vi "add tag to table.vi"(8 "error in":errorcluster, 10 "system tag":refnum<class "tag descriptor.lvclass">, 11 "data table in":T1) -> (0 "error out":errorcluster, 3 "data table out":T1)   [LabVIEW 2013, in "tag bus.lvlib" / "data table.lvlib"]
doc: "Adds a tag to a data table."
uses:
  data table.lvlib
  data table.ctl
  tag/tag descriptor.lvclass
  tag/tag descriptor.lvclass/tag descriptor.ctl
  tag/default value polymorphs/read default value Double.vi
  tag/default value polymorphs/read default value Single.vi
  tag/default value polymorphs/read default value I64.vi
  tag/default value polymorphs/read default value I32.vi
  tag/default value polymorphs/read default value I16.vi
  tag/default value polymorphs/read default value I8.vi
  tag/default value polymorphs/read default value U64.vi
  tag/default value polymorphs/read default value U32.vi
  tag/default value polymorphs/read default value U16.vi
  tag/default value polymorphs/read default value U8.vi
  tag/default value polymorphs/read default value String.vi
  tag/default value polymorphs/read default value Boolean.vi
  tag/default value polymorphs/read default value Array of U8.vi
  tag/default value polymorphs/read default value Array of U16.vi
  tag/default value polymorphs/read default value Array of U32.vi
  tag/default value polymorphs/read default value Array of U64.vi
  tag/default value polymorphs/read default value Array of I64.vi
  tag/default value polymorphs/read default value Array of I32.vi
  tag/default value polymorphs/read default value Array of I16.vi
  tag/default value polymorphs/read default value Array of I8.vi
  tag/default value polymorphs/read default value Array of Double.vi
  tag/default value polymorphs/read default value Array of Single.vi
  tag/default value polymorphs/read default value Array of Boolean.vi
  tag/default value polymorphs/read default value Array of String.vi
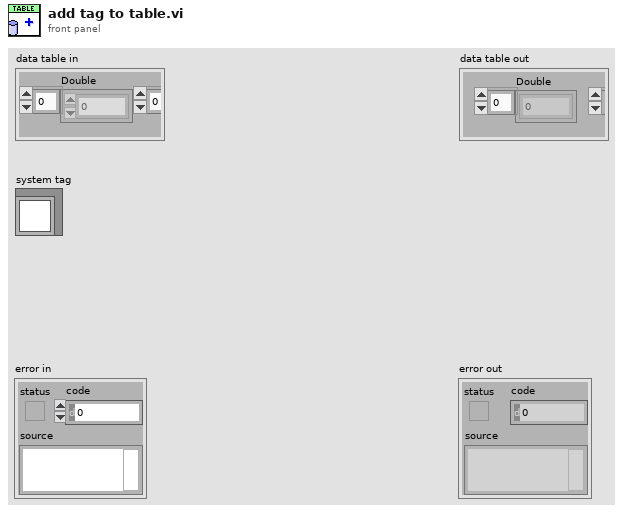
[diagram p1: front panel]
types:
  T1 = typedef "tag bus.lvlib/data table.lvlib/data table.ctl" = cluster{"Double":dbl[], "Single":sgl[], "I64":i64[], "I32":i32[], "I16":i16[], "I8":i8[], "U64":u64[], "U32":u32[], "U16":u16[], "U8":u8[], "Boolean":bool[], "String":string[], "Array of Double":cluster{"DBL Array":dbl[]}[], "Array of Single":cluster{"SGL Array":sgl[]}[], "Array of I64":cluster{"I64 Array":i64[]}[], "Array of I32":cluster{"I32 Array":i32[]}[], "Array of I16":cluster{"I16 Array":i16[]}[], "Array of I8":cluster{"I8 Array":i8[]}[], "Array of U64":cluster{"U64 Array":u64[]}[], "Array of U32":cluster{"U32 Array":u32[]}[], "Array of U16":cluster{"U16 Array":u16[]}[], "Array of U8":cluster{"U8 Array":u8[]}[], "Array of Boolean":cluster{"Boolean Array":bool[]}[], "Array of String":cluster{"String Array":string[]}[]}
  T2 = typedef "tag bus.lvlib/tag descriptor.lvclass/Data Type.ctl" = enum16{"Double", "Single", "I64", "I32", "I16", "I8", "U64", "U32", "U16", "U8", "Boolean", "String", "Array of Double", "Array of Single", "Array of I64", "Array of I32", "Array of I16", "Array of I8", "Array of U64", "Array of U32", "Array of U16", "Array of U8", "Array of Boolean", "Array of String"}
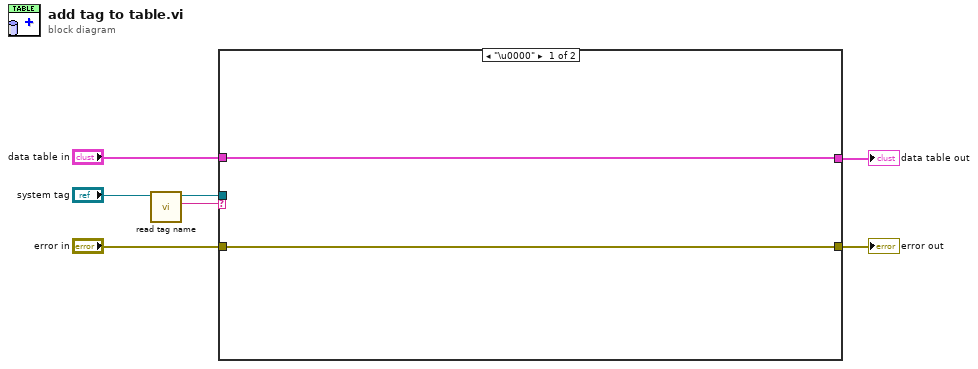
[diagram p0: block diagram]
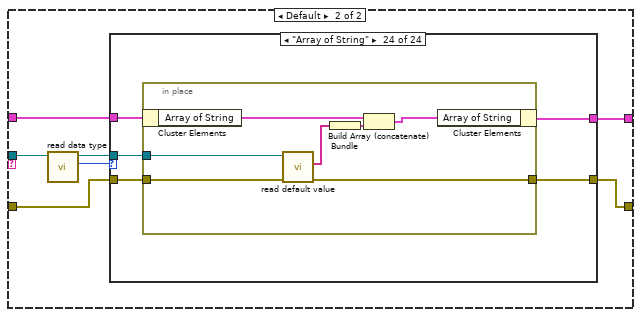
[diagram p2: hidden frame]
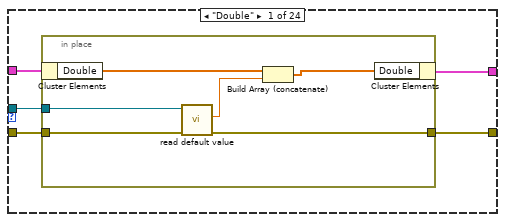
[diagram p3: hidden frame]
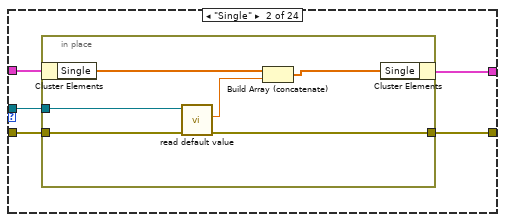
[diagram p4: hidden frame]
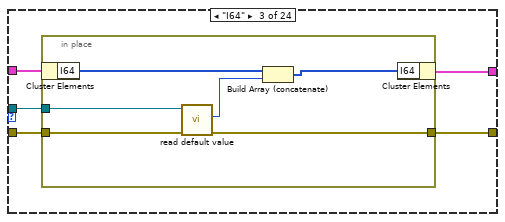
[diagram p5: hidden frame]
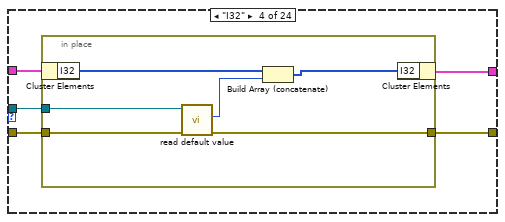
[diagram p6: hidden frame]
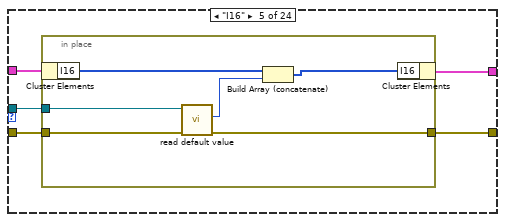
[diagram p7: hidden frame]
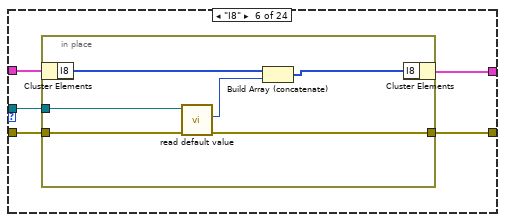
[diagram p8: hidden frame]
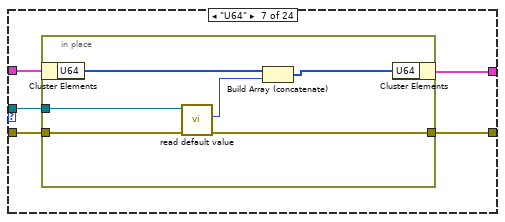
[diagram p9: hidden frame]
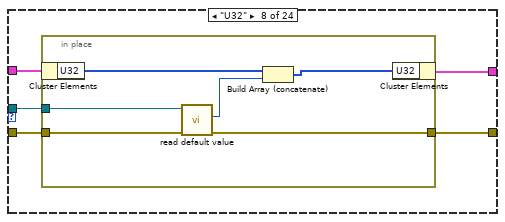
[diagram p10: hidden frame]
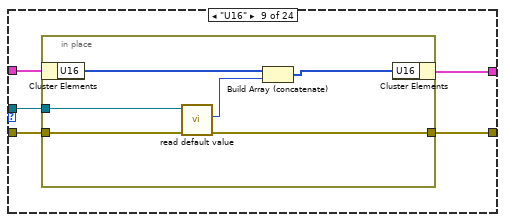
[diagram p11: hidden frame]
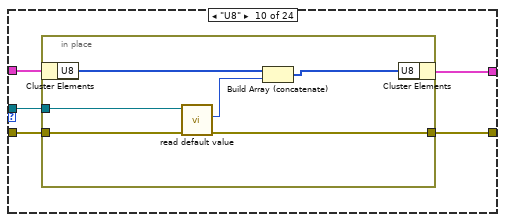
[diagram p12: hidden frame]
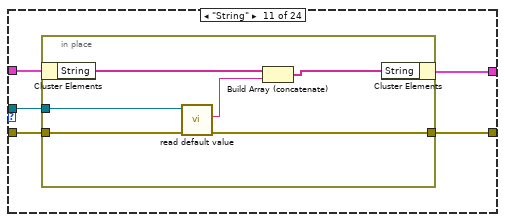
[diagram p13: hidden frame]
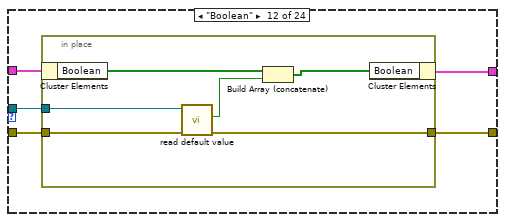
[diagram p14: hidden frame]
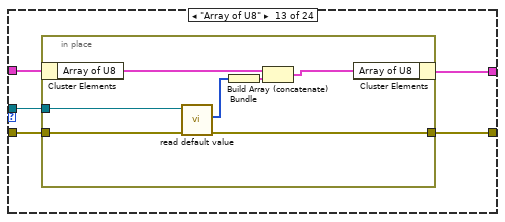
[diagram p15: hidden frame]
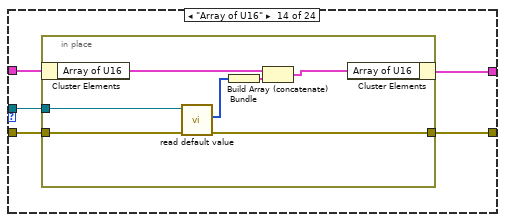
[diagram p16: hidden frame]
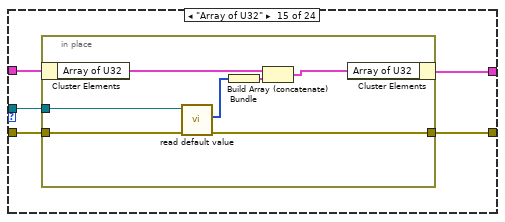
[diagram p17: hidden frame]
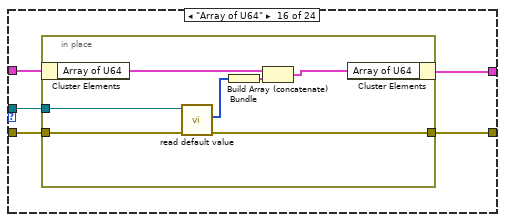
[diagram p18: hidden frame]
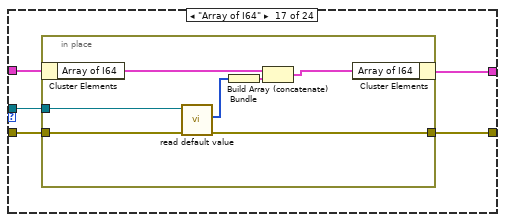
[diagram p19: hidden frame]
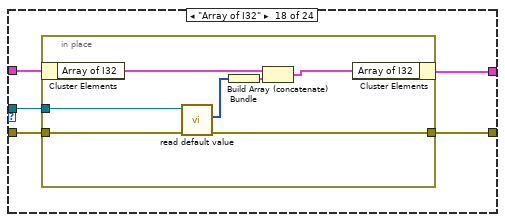
[diagram p20: hidden frame]
diagram:
  n1 = call "read tag name.vi"("system tag in"="system tag") -> ("name"=w1:string, "system tag out"=w2:refnum<class "tag descriptor.lvclass">)  [unwired: 8 in, 1 out]
  n2 = case shown="\"\"" w1 {
    tunnel: "data table in" -> [w9 w15]
    tunnel: [w9 w14] -> w6
    tunnel: "error in" -> [w8 w12]
    tunnel: [w8 w11] -> w4
    tunnel: w2 -> [_ w10]
    frame "\u0000" {
    }
    frame Default {
      n3 = call "read data type.vi"("system tag in"=w10) -> ("data type"=w16:T2, "system tag out"=w13:refnum<class "tag descriptor.lvclass">)  [unwired: 8 in, 1 out]
      n4 = case shown="\"Array of String\"" w16 {
        tunnel: w15 -> [w21 w32 w43 w54 w65 w76 w87 w98 w109 w120 w131 w142 w153 w165 w177 w189 w201 w213 w225 w237 w249 w261 w273 w285]
        tunnel: [w20 w31 w42 w53 w64 w75 w86 w97 w108 w119 w130 w141 w152 w164 w176 w188 w200 w212 w224 w236 w248 w260 w272 w284] -> w14
        tunnel: w13 -> [w19 w30 w41 w52 w63 w74 w85 w96 w107 w118 w129 w140 w151 w163 w175 w187 w199 w211 w223 w235 w247 w259 w271 w283]
        tunnel: w12 -> [w18 w29 w40 w51 w62 w73 w84 w95 w106 w117 w128 w139 w150 w162 w174 w186 w198 w210 w222 w234 w246 w258 w270 w282]
        tunnel: [w17 w28 w39 w50 w61 w72 w83 w94 w105 w116 w127 w138 w149 w161 w173 w185 w197 w209 w221 w233 w245 w257 w269 w281] -> w11
        frame "Double" {
          n5 = in-place {
            in-place-border: w19 -> [w27]
            in-place-border: w18 -> [w24]
            in-place-border: [w22] -> w17
            n6 = in-place-cluster #1(w21) -> ("Double"=w26:dbl[])
            n7 = call-poly "read default value.vi"("error in"=w24, "system tag in"=w27) -> ("error out"=w22:errorcluster, "default value"=w25:dbl)  [unwired: 6 in, 2 out]
            n8 = Build Array (concatenate)(w26, w25) -> (w23:dbl[])
            n9 = in-place-cluster #1("Double"=w23) -> (w20:T1)
          }
        }
        frame "Single" {
          n10 = in-place {
            in-place-border: w30 -> [w38]
            in-place-border: w29 -> [w35]
            in-place-border: [w33] -> w28
            n11 = in-place-cluster #2(w32) -> ("Single"=w37:sgl[])
            n12 = call-poly "read default value.vi"("error in"=w35, "system tag in"=w38) -> ("error out"=w33:errorcluster, "default value"=w36:sgl)  [unwired: 6 in, 2 out]
            n13 = Build Array (concatenate)(w37, w36) -> (w34:sgl[])
            n14 = in-place-cluster #2("Single"=w34) -> (w31:T1)
          }
        }
        frame "I64" {
          n15 = in-place {
            in-place-border: w41 -> [w49]
            in-place-border: w40 -> [w46]
            in-place-border: [w44] -> w39
            n16 = in-place-cluster #3(w43) -> ("I64"=w48:i64[])
            n17 = call-poly "read default value.vi"("error in"=w46, "system tag in"=w49) -> ("error out"=w44:errorcluster, "default value"=w47:i64)  [unwired: 6 in, 2 out]
            n18 = Build Array (concatenate)(w48, w47) -> (w45:i64[])
            n19 = in-place-cluster #3("I64"=w45) -> (w42:T1)
          }
        }
        frame "I32" {
          n20 = in-place {
            in-place-border: w52 -> [w60]
            in-place-border: w51 -> [w57]
            in-place-border: [w55] -> w50
            n21 = in-place-cluster #4(w54) -> ("I32"=w59:i32[])
            n22 = call-poly "read default value.vi"("error in"=w57, "system tag in"=w60) -> ("error out"=w55:errorcluster, "default value"=w58:i32)  [unwired: 6 in, 2 out]
            n23 = Build Array (concatenate)(w59, w58) -> (w56:i32[])
            n24 = in-place-cluster #4("I32"=w56) -> (w53:T1)
          }
        }
        frame "I16" {
          n25 = in-place {
            in-place-border: w63 -> [w71]
            in-place-border: w62 -> [w68]
            in-place-border: [w66] -> w61
            n26 = in-place-cluster #5(w65) -> ("I16"=w70:i16[])
            n27 = call-poly "read default value.vi"("error in"=w68, "system tag in"=w71) -> ("error out"=w66:errorcluster, "default value"=w69:i16)  [unwired: 6 in, 2 out]
            n28 = Build Array (concatenate)(w70, w69) -> (w67:i16[])
            n29 = in-place-cluster #5("I16"=w67) -> (w64:T1)
          }
        }
        frame "I8" {
          n30 = in-place {
            in-place-border: w74 -> [w82]
            in-place-border: w73 -> [w79]
            in-place-border: [w77] -> w72
            n31 = in-place-cluster #6(w76) -> ("I8"=w81:i8[])
            n32 = call-poly "read default value.vi"("error in"=w79, "system tag in"=w82) -> ("error out"=w77:errorcluster, "default value"=w80:i8)  [unwired: 6 in, 2 out]
            n33 = Build Array (concatenate)(w81, w80) -> (w78:i8[])
            n34 = in-place-cluster #6("I8"=w78) -> (w75:T1)
          }
        }
        frame "U64" {
          n35 = in-place {
            in-place-border: w85 -> [w93]
            in-place-border: w84 -> [w90]
            in-place-border: [w88] -> w83
            n36 = in-place-cluster #7(w87) -> ("U64"=w92:u64[])
            n37 = call-poly "read default value.vi"("error in"=w90, "system tag in"=w93) -> ("error out"=w88:errorcluster, "default value"=w91:u64)  [unwired: 6 in, 2 out]
            n38 = Build Array (concatenate)(w92, w91) -> (w89:u64[])
            n39 = in-place-cluster #7("U64"=w89) -> (w86:T1)
          }
        }
        frame "U32" {
          n40 = in-place {
            in-place-border: w96 -> [w104]
            in-place-border: w95 -> [w101]
            in-place-border: [w99] -> w94
            n41 = in-place-cluster #8(w98) -> ("U32"=w103:u32[])
            n42 = call-poly "read default value.vi"("error in"=w101, "system tag in"=w104) -> ("error out"=w99:errorcluster, "default value"=w102:u32)  [unwired: 6 in, 2 out]
            n43 = Build Array (concatenate)(w103, w102) -> (w100:u32[])
            n44 = in-place-cluster #8("U32"=w100) -> (w97:T1)
          }
        }
        frame "U16" {
          n45 = in-place {
            in-place-border: w107 -> [w115]
            in-place-border: w106 -> [w112]
            in-place-border: [w110] -> w105
            n46 = in-place-cluster #9(w109) -> ("U16"=w114:u16[])
            n47 = call-poly "read default value.vi"("error in"=w112, "system tag in"=w115) -> ("error out"=w110:errorcluster, "default value"=w113:u16)  [unwired: 6 in, 2 out]
            n48 = Build Array (concatenate)(w114, w113) -> (w111:u16[])
            n49 = in-place-cluster #9("U16"=w111) -> (w108:T1)
          }
        }
        frame "U8" {
          n50 = in-place {
            in-place-border: w118 -> [w126]
            in-place-border: w117 -> [w123]
            in-place-border: [w121] -> w116
            n51 = in-place-cluster #10(w120) -> ("U8"=w125:u8[])
            n52 = call-poly "read default value.vi"("error in"=w123, "system tag in"=w126) -> ("error out"=w121:errorcluster, "default value"=w124:u8)  [unwired: 6 in, 2 out]
            n53 = Build Array (concatenate)(w125, w124) -> (w122:u8[])
            n54 = in-place-cluster #10("U8"=w122) -> (w119:T1)
          }
        }
        frame "String" {
          n55 = in-place {
            in-place-border: w129 -> [w137]
            in-place-border: w128 -> [w134]
            in-place-border: [w132] -> w127
            n56 = in-place-cluster #11(w131) -> ("String"=w136:string[])
            n57 = call-poly "read default value.vi"("error in"=w134, "system tag in"=w137) -> ("error out"=w132:errorcluster, "default value"=w135:string)  [unwired: 6 in, 2 out]
            n58 = Build Array (concatenate)(w136, w135) -> (w133:string[])
            n59 = in-place-cluster #11("String"=w133) -> (w130:T1)
          }
        }
        frame "Boolean" {
          n60 = in-place {
            in-place-border: w140 -> [w148]
            in-place-border: w139 -> [w145]
            in-place-border: [w143] -> w138
            n61 = in-place-cluster #12(w142) -> ("Boolean"=w147:bool[])
            n62 = call-poly "read default value.vi"("error in"=w145, "system tag in"=w148) -> ("error out"=w143:errorcluster, "default value"=w146:bool)  [unwired: 6 in, 2 out]
            n63 = Build Array (concatenate)(w147, w146) -> (w144:bool[])
            n64 = in-place-cluster #12("Boolean"=w144) -> (w141:T1)
          }
        }
        frame "Array of U8" {
          n65 = in-place {
            in-place-border: w151 -> [w160]
            in-place-border: w150 -> [w157]
            in-place-border: [w155] -> w149
            n66 = in-place-cluster #13(w153) -> ("Array of U8"=w159:cluster{"U8 Array":u8[]}[])
            n67 = call-poly "read default value.vi"("error in"=w157, "system tag in"=w160) -> ("error out"=w155:errorcluster, "default value"=w158:u8[])  [unwired: 6 in, 2 out]
            n68 = Bundle("default value"=w158) -> (w154:cluster{"default value":u8[]})  [unwired: 1 in]
            n69 = Build Array (concatenate)(w159, w154) -> (w156:cluster{"default value":u8[]}[])
            n70 = in-place-cluster #13("Array of U8"=w156) -> (w152:T1)
          }
        }
        frame "Array of U16" {
          n71 = in-place {
            in-place-border: w163 -> [w172]
            in-place-border: w162 -> [w169]
            in-place-border: [w167] -> w161
            n72 = in-place-cluster #14(w165) -> ("Array of U16"=w171:cluster{"U16 Array":u16[]}[])
            n73 = call-poly "read default value.vi"("error in"=w169, "system tag in"=w172) -> ("error out"=w167:errorcluster, "default value"=w170:u16[])  [unwired: 6 in, 2 out]
            n74 = Bundle("default value"=w170) -> (w166:cluster{"default value":u16[]})  [unwired: 1 in]
            n75 = Build Array (concatenate)(w171, w166) -> (w168:cluster{"default value":u16[]}[])
            n76 = in-place-cluster #14("Array of U16"=w168) -> (w164:T1)
          }
        }
        frame "Array of U32" {
          n77 = in-place {
            in-place-border: w175 -> [w184]
            in-place-border: w174 -> [w181]
            in-place-border: [w179] -> w173
            n78 = in-place-cluster #15(w177) -> ("Array of U32"=w183:cluster{"U32 Array":u32[]}[])
            n79 = call-poly "read default value.vi"("error in"=w181, "system tag in"=w184) -> ("error out"=w179:errorcluster, "default value"=w182:u32[])  [unwired: 6 in, 2 out]
            n80 = Bundle("default value"=w182) -> (w178:cluster{"default value":u32[]})  [unwired: 1 in]
            n81 = Build Array (concatenate)(w183, w178) -> (w180:cluster{"default value":u32[]}[])
            n82 = in-place-cluster #15("Array of U32"=w180) -> (w176:T1)
          }
        }
        frame "Array of U64" {
          n83 = in-place {
            in-place-border: w187 -> [w196]
            in-place-border: w186 -> [w193]
            in-place-border: [w191] -> w185
            n84 = in-place-cluster #16(w189) -> ("Array of U64"=w195:cluster{"U64 Array":u64[]}[])
            n85 = call-poly "read default value.vi"("error in"=w193, "system tag in"=w196) -> ("error out"=w191:errorcluster, "default value"=w194:u64[])  [unwired: 6 in, 2 out]
            n86 = Bundle("default value"=w194) -> (w190:cluster{"default value":u64[]})  [unwired: 1 in]
            n87 = Build Array (concatenate)(w195, w190) -> (w192:cluster{"default value":u64[]}[])
            n88 = in-place-cluster #16("Array of U64"=w192) -> (w188:T1)
          }
        }
        frame "Array of I64" {
          n89 = in-place {
            in-place-border: w199 -> [w208]
            in-place-border: w198 -> [w205]
            in-place-border: [w203] -> w197
            n90 = in-place-cluster #17(w201) -> ("Array of I64"=w207:cluster{"I64 Array":i64[]}[])
            n91 = call-poly "read default value.vi"("error in"=w205, "system tag in"=w208) -> ("error out"=w203:errorcluster, "default value"=w206:i64[])  [unwired: 6 in, 2 out]
            n92 = Bundle("default value"=w206) -> (w202:cluster{"default value":i64[]})  [unwired: 1 in]
            n93 = Build Array (concatenate)(w207, w202) -> (w204:cluster{"default value":i64[]}[])
            n94 = in-place-cluster #17("Array of I64"=w204) -> (w200:T1)
          }
        }
        frame "Array of I32" {
          n95 = in-place {
            in-place-border: w211 -> [w220]
            in-place-border: w210 -> [w217]
            in-place-border: [w215] -> w209
            n96 = in-place-cluster #18(w213) -> ("Array of I32"=w219:cluster{"I32 Array":i32[]}[])
            n97 = call-poly "read default value.vi"("error in"=w217, "system tag in"=w220) -> ("error out"=w215:errorcluster, "default value"=w218:i32[])  [unwired: 6 in, 2 out]
            n98 = Bundle("default value"=w218) -> (w214:cluster{"default value":i32[]})  [unwired: 1 in]
            n99 = Build Array (concatenate)(w219, w214) -> (w216:cluster{"default value":i32[]}[])
            n100 = in-place-cluster #18("Array of I32"=w216) -> (w212:T1)
          }
        }
        frame "Array of I16" {
          n101 = in-place {
            in-place-border: w223 -> [w232]
            in-place-border: w222 -> [w229]
            in-place-border: [w227] -> w221
            n102 = in-place-cluster #19(w225) -> ("Array of I16"=w231:cluster{"I16 Array":i16[]}[])
            n103 = call-poly "read default value.vi"("error in"=w229, "system tag in"=w232) -> ("error out"=w227:errorcluster, "default value"=w230:i16[])  [unwired: 6 in, 2 out]
            n104 = Bundle("default value"=w230) -> (w226:cluster{"default value":i16[]})  [unwired: 1 in]
            n105 = Build Array (concatenate)(w231, w226) -> (w228:cluster{"default value":i16[]}[])
            n106 = in-place-cluster #19("Array of I16"=w228) -> (w224:T1)
          }
        }
        frame "Array of I8" {
          n107 = in-place {
            in-place-border: w235 -> [w244]
            in-place-border: w234 -> [w241]
            in-place-border: [w239] -> w233
            n108 = in-place-cluster #20(w237) -> ("Array of I8"=w243:cluster{"I8 Array":i8[]}[])
            n109 = call-poly "read default value.vi"("error in"=w241, "system tag in"=w244) -> ("error out"=w239:errorcluster, "default value"=w242:i8[])  [unwired: 6 in, 2 out]
            n110 = Bundle("default value"=w242) -> (w238:cluster{"default value":i8[]})  [unwired: 1 in]
            n111 = Build Array (concatenate)(w243, w238) -> (w240:cluster{"default value":i8[]}[])
            n112 = in-place-cluster #20("Array of I8"=w240) -> (w236:T1)
          }
        }
        frame "Array of Double" {
          n113 = in-place {
            in-place-border: w247 -> [w256]
            in-place-border: w246 -> [w253]
            in-place-border: [w251] -> w245
            n114 = in-place-cluster #21(w249) -> ("Array of Double"=w255:cluster{"DBL Array":dbl[]}[])
            n115 = call-poly "read default value.vi"("error in"=w253, "system tag in"=w256) -> ("error out"=w251:errorcluster, "default value"=w254:dbl[])  [unwired: 6 in, 2 out]
            n116 = Bundle("default value"=w254) -> (w250:cluster{"default value":dbl[]})  [unwired: 1 in]
            n117 = Build Array (concatenate)(w255, w250) -> (w252:cluster{"default value":dbl[]}[])
            n118 = in-place-cluster #21("Array of Double"=w252) -> (w248:T1)
          }
        }
        frame "Array of Single" {
          n119 = in-place {
            in-place-border: w259 -> [w268]
            in-place-border: w258 -> [w265]
            in-place-border: [w263] -> w257
            n120 = in-place-cluster #22(w261) -> ("Array of Single"=w267:cluster{"SGL Array":sgl[]}[])
            n121 = call-poly "read default value.vi"("error in"=w265, "system tag in"=w268) -> ("error out"=w263:errorcluster, "default value"=w266:sgl[])  [unwired: 6 in, 2 out]
            n122 = Bundle("default value"=w266) -> (w262:cluster{"default value":sgl[]})  [unwired: 1 in]
            n123 = Build Array (concatenate)(w267, w262) -> (w264:cluster{"default value":sgl[]}[])
            n124 = in-place-cluster #22("Array of Single"=w264) -> (w260:T1)
          }
        }
        frame "Array of Boolean" {
          n125 = in-place {
            in-place-border: w271 -> [w280]
            in-place-border: w270 -> [w277]
            in-place-border: [w275] -> w269
            n126 = in-place-cluster #23(w273) -> ("Array of Boolean"=w279:cluster{"Boolean Array":bool[]}[])
            n127 = call-poly "read default value.vi"("error in"=w277, "system tag in"=w280) -> ("error out"=w275:errorcluster, "default value"=w278:bool[])  [unwired: 6 in, 2 out]
            n128 = Bundle("default value"=w278) -> (w274:cluster{"default value":bool[]})  [unwired: 1 in]
            n129 = Build Array (concatenate)(w279, w274) -> (w276:cluster{"default value":bool[]}[])
            n130 = in-place-cluster #23("Array of Boolean"=w276) -> (w272:T1)
          }
        }
        frame "Array of String" {
          n131 = in-place {
            in-place-border: w283 -> [w292]
            in-place-border: w282 -> [w289]
            in-place-border: [w287] -> w281
            n132 = in-place-cluster #24(w285) -> ("Array of String"=w291:cluster{"String Array":string[]}[])
            n133 = call-poly "read default value.vi"("error in"=w289, "system tag in"=w292) -> ("error out"=w287:errorcluster, "default value"=w290:string[])  [unwired: 6 in, 2 out]
            n134 = Bundle("default value"=w290) -> (w286:cluster{"default value":string[]})  [unwired: 1 in]
            n135 = Build Array (concatenate)(w291, w286) -> (w288:cluster{"default value":string[]}[])
            n136 = in-place-cluster #24("Array of String"=w288) -> (w284:T1)
          }
        }
      }
    }
  }
  "error out" <- w4
  "data table out" <- w6
